vi "Parse Sysdef.vi"(0 "Device Reference in":T6 format="%.0x", 1 "rx channel handle array":u32[](array[numeric]), 3 "tx channel handle array":u32[](array[numeric]), 5 "error in (no error)":errorcluster, 7 "FIFO Idx Qs":T5) -> (6 "Status Config":T4 {"HWOut Dur Ref" format="%.0x"; "HWIn Dur Ref" format="%.0x"; "Error Data Ref" format="%.0x"}, 8 "ScheduledSDI":bool, 10 "HWIn BaseRate":i32, 12 "HWOut BaseRate":i32, 14 "Device Reference out":T6 format="%.0x", 15 "HWOutput Section Data":T7[](array[typedef]) {"Labels Settings"."Label" format="%.0o"}, 17 "HWInput Section Data":T7[](array[typedef]) {"Labels Settings"."Label" format="%.0o"}, 18 "Label Transfer Config":T1 {"Block Data Refs"."Data Reference" format="%.0x"}, 19 "error out":errorcluster)   [LabVIEW 2012, in "AIT 429 Custom Device.lvlib"]
uses:
  AIT 429 Custom Device.lvlib
  Controls and Global/Global.vi
  <vilib>/NI Veristand/Custom Device API/Data Access Type.ctl
  <vilib>/NI Veristand/Custom Device API/Custom Device API.lvlib
  <vilib>/NI Veristand/Custom Device API/Get Item Property (Boolean).vi
  Controls and Global/Label.ctl
  Controls and Global/transferPeriod.ctl
  <vilib>/NI Veristand/Custom Device API/Data Reference.ctl
  <vilib>/NI Veristand/Custom Device API/Block Data Reference.ctl
  Controls and Global/Start Bit.ctl
  Controls and Global/Number of Bits.ctl
  RT Controls/RT Label Settings.ctl
  RT Controls/RT HW Channel.ctl
  <vilib>/NI Veristand/Custom Device API/Custom Device Item Ref.ctl
  RT Controls/Driver Data.ctl
  RT Controls/FIFO Idx Qs.ctl
  RT Controls/Status Channels Config.ctl
  RT Controls/Label Transfer Config.ctl
  RT Controls/RT Param Setting.ctl
  RT Controls/RT Word Settings.ctl
  Controls and Global/TransferType.ctl
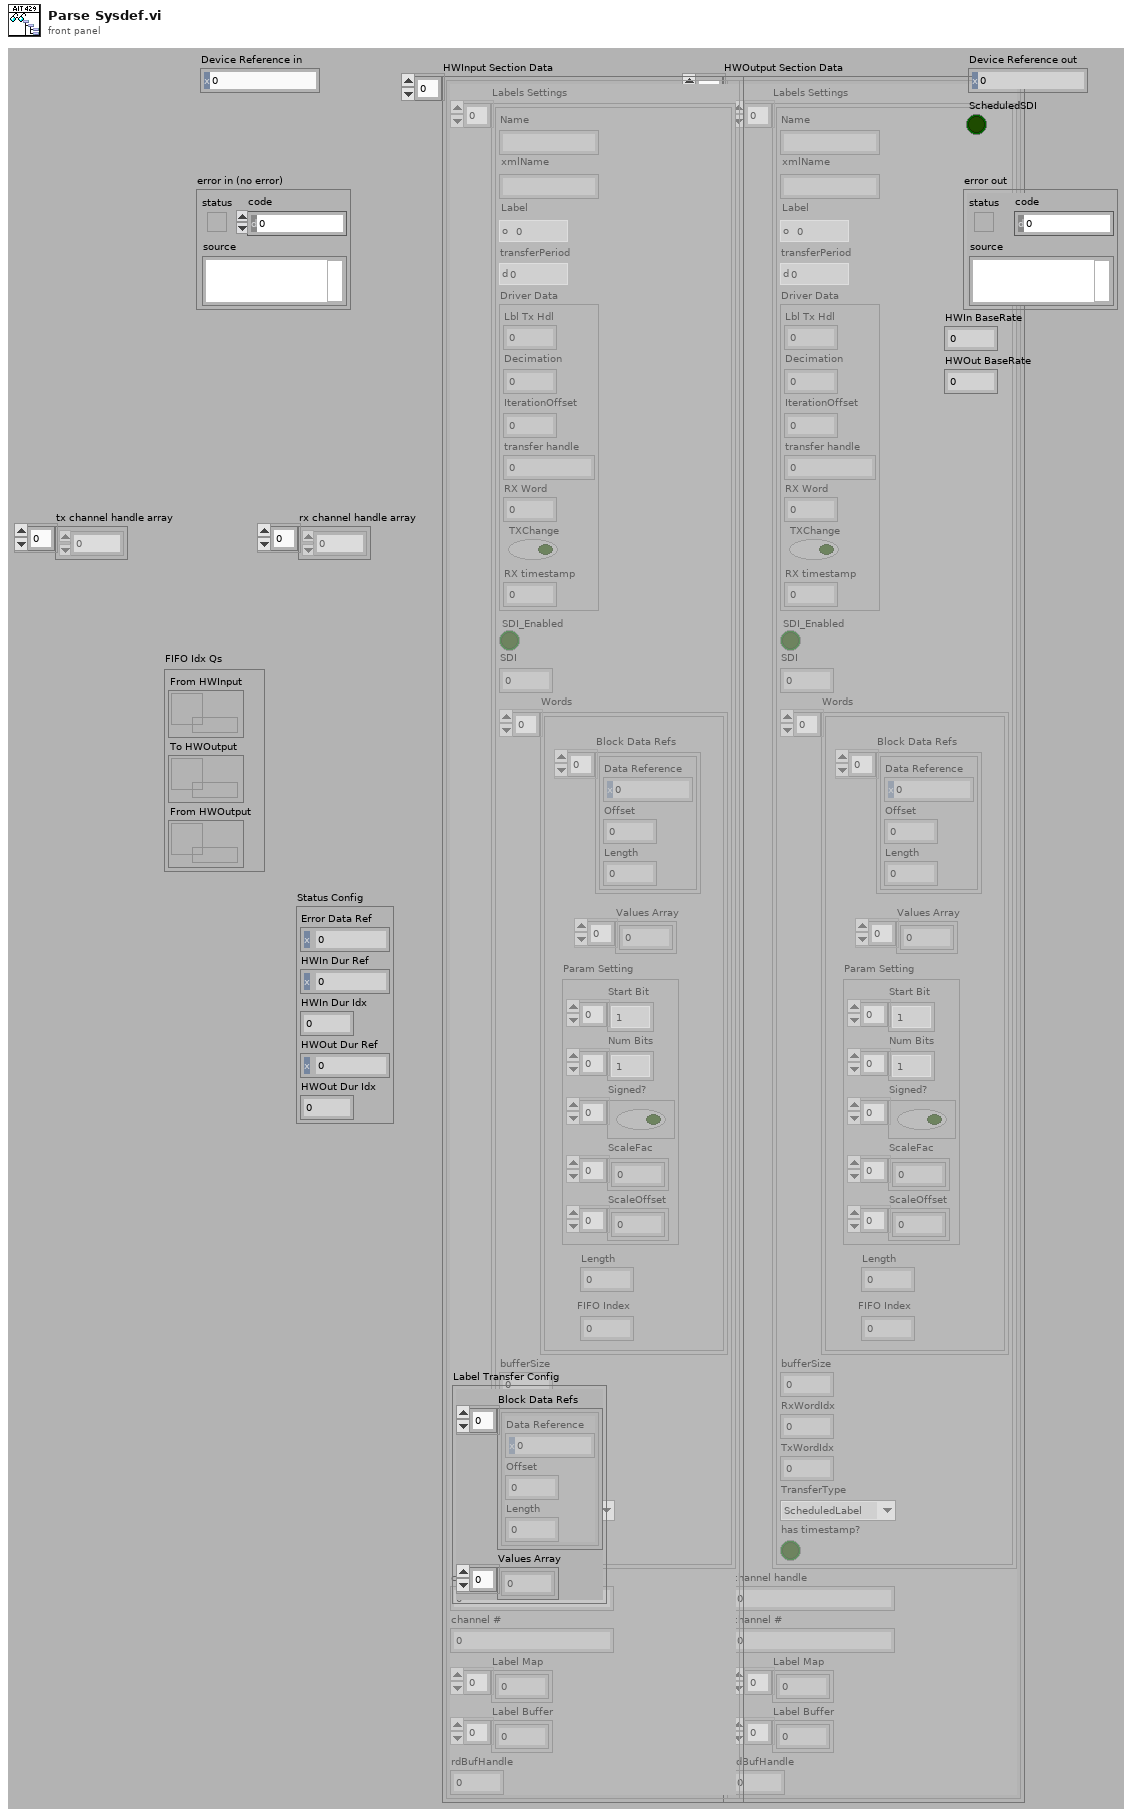
[diagram p1: front panel]
types:
  T1 = typedef "AIT 429 Custom Device.lvlib/Label Transfer Config.ctl" = cluster{"Block Data Refs":T2[], "Values Array":dbl[]}
  T2 = typedef "Custom Device API.lvlib/Block Data Reference.ctl" = cluster{"Data Reference":T3, "Offset":i32, "Length":i32}
  T3 = typedef "Custom Device API.lvlib/Data Reference.ctl" = i32
  T4 = typedef "AIT 429 Custom Device.lvlib/Status Channels Config.ctl" = cluster{"Error Data Ref":T3, "HWIn Dur Ref":T3, "HWIn Dur Idx":i32, "HWOut Dur Ref":T3, "HWOut Dur Idx":i32}
  T5 = typedef "AIT 429 Custom Device.lvlib/FIFO Idx Qs.ctl" = cluster{"From HWInput":refnum<queue>, "To HWOutput":refnum<queue>, "From HWOutput":refnum<queue>}
  T6 = typedef "Custom Device API.lvlib/Custom Device Item Ref.ctl" = u64
  T7 = typedef "AIT 429 Custom Device.lvlib/RT HW Channel.ctl" = cluster{"Labels Settings":T8[], "channel handle":u32, "channel #":u16, "Label Map":i32[], "Label Buffer":u32[], "rdBufHandle":u32}
  T8 = typedef "AIT 429 Custom Device.lvlib/RT Label Settings.ctl" = cluster{"Name":string, "xmlName":string, "Label":T9, "transferPeriod":T10, "Driver Data":T11, "SDI_Enabled":bool, "SDI":u8, "Words":T12[], "bufferSize":u32, "RxWordIdx":i32, "TxWordIdx":i32, "TransferType":T16, "has timestamp?":bool}
  T9 = typedef "AIT 429 Custom Device.lvlib/Label.ctl" = u8
  T10 = typedef "AIT 429 Custom Device.lvlib/transferPeriod.ctl" = u32
  T11 = typedef "AIT 429 Custom Device.lvlib/Driver Data.ctl" = cluster{"Lbl Tx Hdl":u32, "Decimation":i32, "IterationOffset":i32, "transfer handle":u32, "RX Word":u32, "TXChange":bool, "RX timestamp":dbl}
  T12 = typedef "AIT 429 Custom Device.lvlib/RT Word Settings.ctl" = cluster{"Block Data Refs":T2[], "Values Array":dbl[], "Length":i32, "FIFO Index":i32, "Param Setting":T13}
  T13 = typedef "AIT 429 Custom Device.lvlib/Rt Param Setting.ctl" = cluster{"Start Bit":T14[], "Num Bits":T15[], "Signed?":bool[], "ScaleFac":dbl[], "ScaleOffset":dbl[]}
  T14 = typedef "AIT 429 Custom Device.lvlib/Start Bit.ctl" = i32
  T15 = typedef "AIT 429 Custom Device.lvlib/Number of Bits.ctl" = i32
  T16 = typedef "AIT 429 Custom Device.lvlib/TransferType.ctl" = enum16{"ScheduledLabel", "Acyclic", "Block", "Strobe"}
  T17 = typedef "Custom Device API.lvlib/Data Access Type.ctl" = enum16{"Read", "Write"}
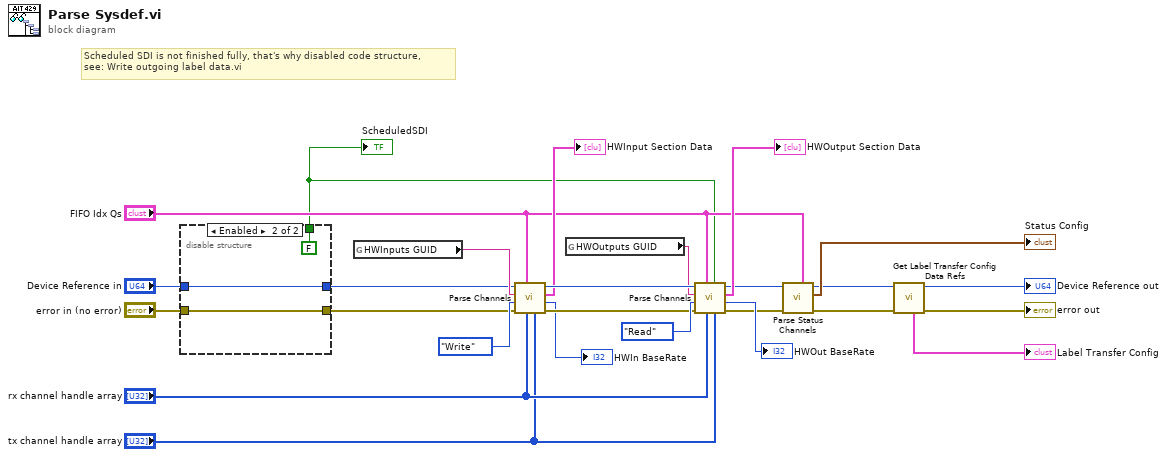
[diagram p0: block diagram]
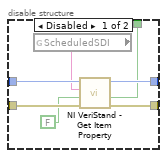
[diagram p2: hidden frame]
diagram:
  # "Scheduled SDI is not finished fully, that's why disabled code structure, \nsee: Write outgoing label data.vi"
  n1 = disable-structure shown="Enabled" {
    disable-tunnel: "Device Reference in" -> [w33 w36]
    disable-tunnel: [w32 w36] -> w4
    disable-tunnel: "error in (no error)" -> [w31 w35]
    disable-tunnel: [w30 w35] -> w2
    disable-tunnel: [w29 FALSE ("ScheduledSDI")] -> w1
    frame Disabled {
      n2 = global read "Global.vi" "ScheduledSDI"() -> (w28:string)
      n3 = call-poly <vilib>:"NI VeriStand - Get Item Property.vi"("error in (no error)"=w31, "Default Value"=FALSE, "Property Name"=w28, "Item Ref in"=w33) -> ("error out"=w30:errorcluster, "Value"=w29:bool, "Item Ref out"=w32:T6)  [unwired: 4 in, 1 out]
    }
    frame Enabled {
    }
  }
  "ScheduledSDI" <- w1
  n4 = global read "Global.vi" "HWInputs GUID"() -> (w21:string)
  n5 = call "Parse Channels.vi"("tx channel handle array"="tx channel handle array", "rx channel handle array"="rx channel handle array", "FIFO Idx Qs"="FIFO Idx Qs", "error in (no error)"=w2, "Access"=Data_Access_Type."Write", "Section GUID"=w21, "Device Reference in"=w4) -> ("error out"=w23:errorcluster, "Section BaseRate"=→"HWIn BaseRate":i32, "Section Data"=→"HWInput Section Data":T7[], "Device Reference out"=w25:T6)  [unwired: 1 in]
  n6 = global read "Global.vi" "HWOutputs GUID"() -> (w24:string)
  n7 = call "Parse Channels.vi"("tx channel handle array"="tx channel handle array", "ScheduledSDI"=w1, "rx channel handle array"="rx channel handle array", "FIFO Idx Qs"="FIFO Idx Qs", "error in (no error)"=w23, "Access"=Data_Access_Type."Read", "Section GUID"=w24, "Device Reference in"=w25) -> ("error out"=w15:errorcluster, "Section BaseRate"=→"HWOut BaseRate":i32, "Section Data"=→"HWOutput Section Data":T7[], "Device Reference out"=w16:T6)
  n8 = call "Parse Status Channels.vi"("FIFO Idx Qs"="FIFO Idx Qs", "error in"=w15, "Device Reference in"=w16) -> ("error out"=w11:errorcluster, "Status Config"=→"Status Config":T4, "Device Ref out"=w12:T6)  [unwired: 6 in]
  n9 = call "Get Label Transfer Config Data Refs.vi"("error in"=w11, "Device Ref in"=w12) -> ("error out"=→"error out":errorcluster, "Device Ref out"=→"Device Reference out":T6, "Label Transfer Config"=→"Label Transfer Config":T1)  [unwired: 7 in]
